vi "GenerateTrendReport.vi"(8 "error in (no error)":errorcluster, 10 "ReportSelection":u16) -> (0 "error out":errorcluster, 1 "ExcelError":bool, 3 "ReportPath":path)   [LabVIEW 2013, in "main.lvlib"]
uses:
  main.lvlib
  Globals/DataPathGlobalVariable.vi
  <userlib>/Excel/excel.llb/excel open (path).vi
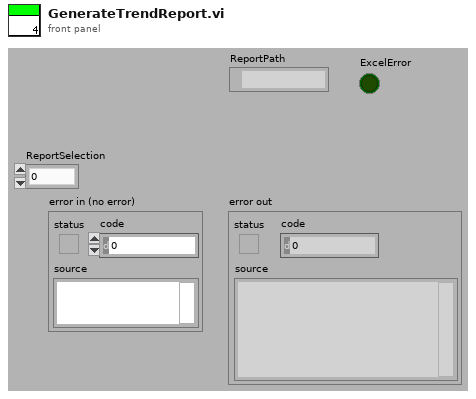
[diagram p1: front panel]
types:
  T1 = cluster{"Palpation":string[], "Personal Info":string[], "Hospital":string[]}
  T2 = enum16{"open workbook as template", "open workbook from file", "create new workbook"}
  T3 = typedef "excel Object Reference.ctl" = refnum<k1>
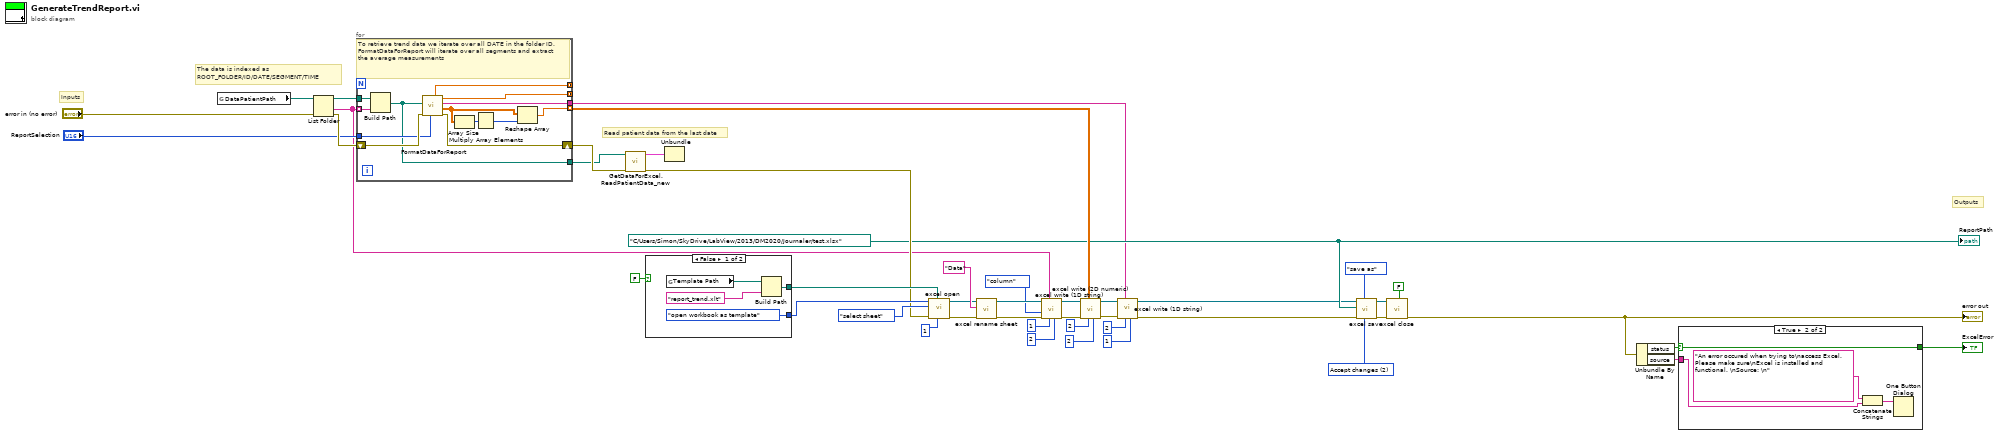
[diagram p0: block diagram]
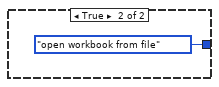
[diagram p2: hidden frame]
diagram:
  w10 = path "C:/Users/Simon/SkyDrive/LabView/2013/DM2020/Journaler/test.xlsx"
  w21 = u16 2 items=["Prompt for changes"=1, "Accept changes"=2, "Reject changes"=3] ("Save As options")
  # "Inputs"
  # "Outputs"
  # "The data is indexed as \nROOT_FOLDER/ID/DATE/SEGMENT/TIME"
  # "Read patient data from the last date"
  n1 = global read "DataPathGlobalVariable.vi" "DataPatientPath"() -> (w42:path)
  n2 = List Folder(path=w42, error in="error in (no error)") -> (path out=w36:path, folder names=w12:string[], error out=w40:errorcluster)  [unwired: 2 in, 1 out]
  n3 = for {
    tunnel: w36 -> [w58]
    tunnel: w12 -> [w57] mode=indexing
    tunnel: "ReportSelection" -> [w55]
    shift-right: [w54] -> w38
    shift-left: w40 -> [w56]
    tunnel: [w53] -> _ mode=concatenating
    tunnel: [w52] -> _ mode=concatenating
    tunnel: [w51] -> w5
    tunnel: [w49] -> w26 mode=indexing
    tunnel: [w50] -> w37
    # "To retrieve trend data we iterate over all DATE in the folder ID. FormatDataForReport will iterate over all segments and extract the average measurements"
    n4 = Build Path(base path=w58, name or relative path=w57) -> (appended path=w50:path)
    n5 = call "FormatDataForReport.vi"("Report selection"=w55, "error in (no error)"=w56, "Path"=w50) -> ("error out"=w54:errorcluster, "Data"=w48:dbl[][], "Names"=w51:string[], "Activity armpressure"=w52:dbl[], "Normal armpressure"=w53:dbl[])  [unwired: 3 in, 1 out]
    n6 = Array Size(array=w48) -> (size(s)=w47:i32[])
    n7 = Multiply Array Elements(1:w47) -> (0:w46:i32)
    n8 = Reshape Array(w48, w46) -> (w49:dbl[])
  }
  n9 = call "GetDataForExcel.ReadPatientData_new.vi"("error in"=w38, "Path"=w37) -> ("error out"=w25:errorcluster, "output cluster"=w44:T1)  [unwired: 8 in]
  n10 = case shown="False" FALSE {
    tunnel: [T2."open workbook as template" ("create/open template/open file") T2."open workbook from file" ("create/open template/open file")] -> w28
    tunnel: [w61 _] -> w29
    frame False {
      n11 = global read "DataPathGlobalVariable.vi" "Template Path"() -> (w60:path)
      n12 = Build Path(base path=w60, name or relative path="report_trend.xlt") -> (appended path=w61:path)
    }
    frame True {
    }
  }
  n13 = Unbundle(w44) -> ()  [unwired: 3 out]
  n14 = call-poly <userlib>:"excel open.vi"("worksheet_number"=u8 1, "workbook path"=w29, "error in (no error)"=w25, "select/new"=enum16{"new sheet", "select sheet"}."select sheet", "create/open template/open file"=w28) -> ("error out"=w30:errorcluster, "reference"=w31:T3)  [unwired: 5 in]
  n15 = call <userlib>:"excel rename sheet.vi"("error in (no error)"=w30, "new name"="Data", "reference"=w31) -> ("error out"=w17:errorcluster, "duplicate reference"=w18:T3)  [unwired: 5 in, 2 out]
  n16 = call <userlib>:"excel write (1D string).vi"("Column"=u32 2, "Row"=u32 1, "1D string array"=w12, "error in (no error)"=w17, "Write array by (row)"=enum16{"row", "column"}."column", "reference"=w18) -> ("error out"=w16:errorcluster, "duplicate reference"=w15:T3)  [unwired: 4 in]
  n17 = call <userlib>:"excel write (2D numeric).vi"("Column"=u32 2, "Row"=u32 2, "2D nurmeric array"=w26, "error in (no error)"=w16, "reference"=w15) -> ("error out"=w8:errorcluster, "duplicate reference"=w9:T3)  [unwired: 5 in]
  n18 = call <userlib>:"excel write (1D string).vi"("Column"=u32 1, "Row"=u32 2, "1D string array"=w5, "error in (no error)"=w8, "reference"=w9) -> ("error out"=w3:errorcluster, "duplicate reference"=w4:T3)  [unwired: 5 in]
  n19 = call <userlib>:"excel save.vi"("Save As options"=w21, "mode (save)"=enum16{"save", "save as", "save a copy as"}."save as", "error in (no error)"=w3, "Path"=w10, "reference"=w4) -> ("error out"=w23:errorcluster, "duplicate reference"=w24:T3)  [unwired: 5 in]
  n20 = call <userlib>:"excel close.vi"("Close"=FALSE, "error in (no error)"=w23, "reference"=w24) -> ("error out"=w11:errorcluster)  [unwired: 8 in]
  "error out" <- w11
  n21 = Unbundle By Name(w11) -> ("status"=w35:bool, "source"=w43:string)
  n22 = case shown="True" w35 {
    selector: w35 -> [w64 w68]
    tunnel: [w64 w68] -> w45
    tunnel: w43 -> [_ w65]
    frame False {
    }
    frame True {
      n23 = Concatenate Strings("An error occured when trying to\naccess Excel. Please make sure\nExcel is installed and functional. \nSource: \n" ("message"), w65) -> (w66:string)
      n24 = One Button Dialog(message=w66) -> ()  [unwired: 1 in, 1 out]
    }
  }
  "ExcelError" <- w45
  "ReportPath" <- w10
